vi "CalcTorqueFromJoint.vi"(8 "error in (no error)":errorcluster, 11 "CAlexData2 in":refnum<class "CAlex2_Data.lvclass">) -> (0 "error out":errorcluster, 1 "AverageTorque":T1, 2 "Torques":T2, 3 "CarexMData out":refnum<class "CAlex2_Data.lvclass">, 4 "Jacobian for Cables":dbl[][](array[numeric]))   [LabVIEW 2016, in "CAlex2_Data.lvclass"]
uses:
  CAlex2-Data/CAlex2_Data.lvclass
  C:/Users/Rand/Desktop/Bilateral-controller/CAlex2-controller/Sim&Process/DataProcess/ExpData/ExpData.lvclass
  <vilib>/Analysis/3filter.llb/Filter Passband Type.ctl
  CAlex2-Data/CAlex2_Data.lvclass/CAlex2_Data.ctl
  <vilib>/Analysis/baseanly.llb/A x Vector.vi
  Classes/CAlex2/CAlex2.lvclass
  C:/Users/Rand/Desktop/Bilateral-controller/CAlex2-controller/Classes/SerialChain/SerialChain.lvclass
  C:/Users/Rand/Desktop/Bilateral-controller/CAlex2-controller/Classes/SerialChain-Cable/SerialChain-Cable.lvclass
  Classes/SerialChain/SerialChain.lvclass
  Classes/SerialChain-Cable/SerialChain-Cable.lvclass
  <vilib>/Analysis/NI_AALBase.lvlib
  ExpData/ExpData.lvclass
  <vilib>/AuZn/auzn custom VIs/AuZnCustomVI.lvlib
panel:
  out "Numeric":i32
  out "PlannedTorque":dbl[][](array[numeric])
  out "ActualTorque":dbl[][](array[numeric])
  out "DesiredTorque":dbl[][](array[numeric])
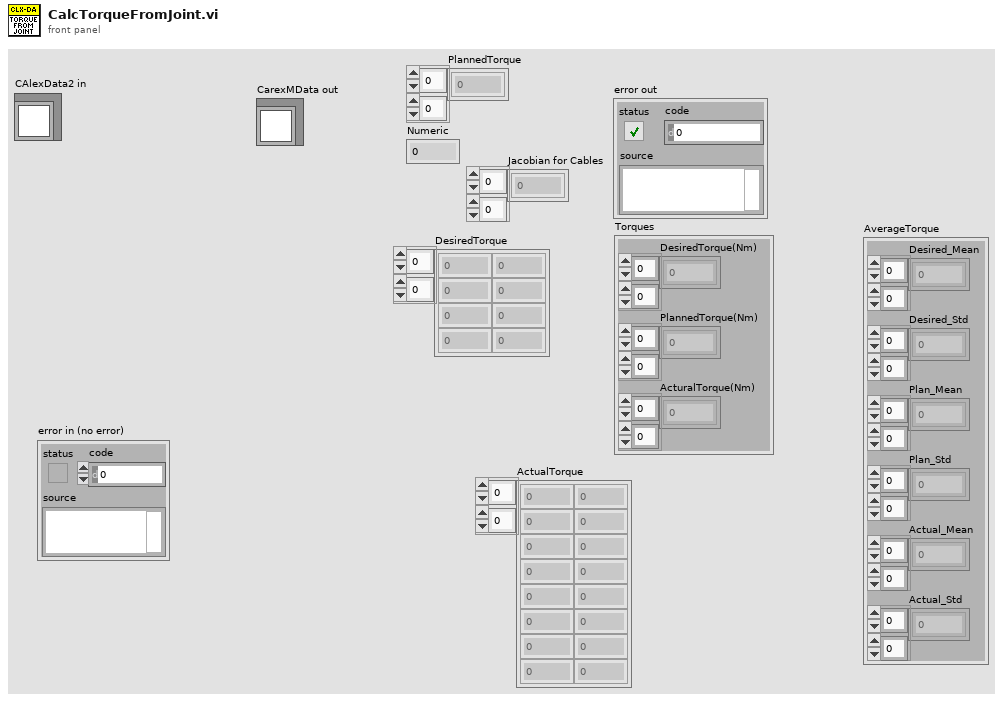
[diagram p1: front panel]
types:
  T1 = cluster{"Desired_Mean":dbl[][], "Desired_Std":dbl[][], "Plan_Mean":dbl[][], "Plan_Std":dbl[][], "Actual_Mean":dbl[][], "Actual_Std":dbl[][]}
  T2 = cluster{"DesiredTorque(Nm)":dbl[][], "PlannedTorque(Nm)":dbl[][], "ActuralTorque(Nm)":dbl[][]}
  T3 = typedef "NI_AALBase.lvlib/Filter Passband Type.ctl" = enum32{"Lowpass", "Highpass", "Bandpass", "Bandstop"}
  T4 = typedef "SerialChain.lvclass/PointOnBody.ctl" = cluster{"Coord4":dbl[], "ID":i32}
  T5 = typedef "NI_Matrix.lvlib/RealMatrix.ctl" = dbl[][]
  T6 = cluster{"Mean":dbl[][], "Std":dbl[][], "Mean":dbl[][], "Std":dbl[][], "Mean":dbl[][], "Std":dbl[][]}
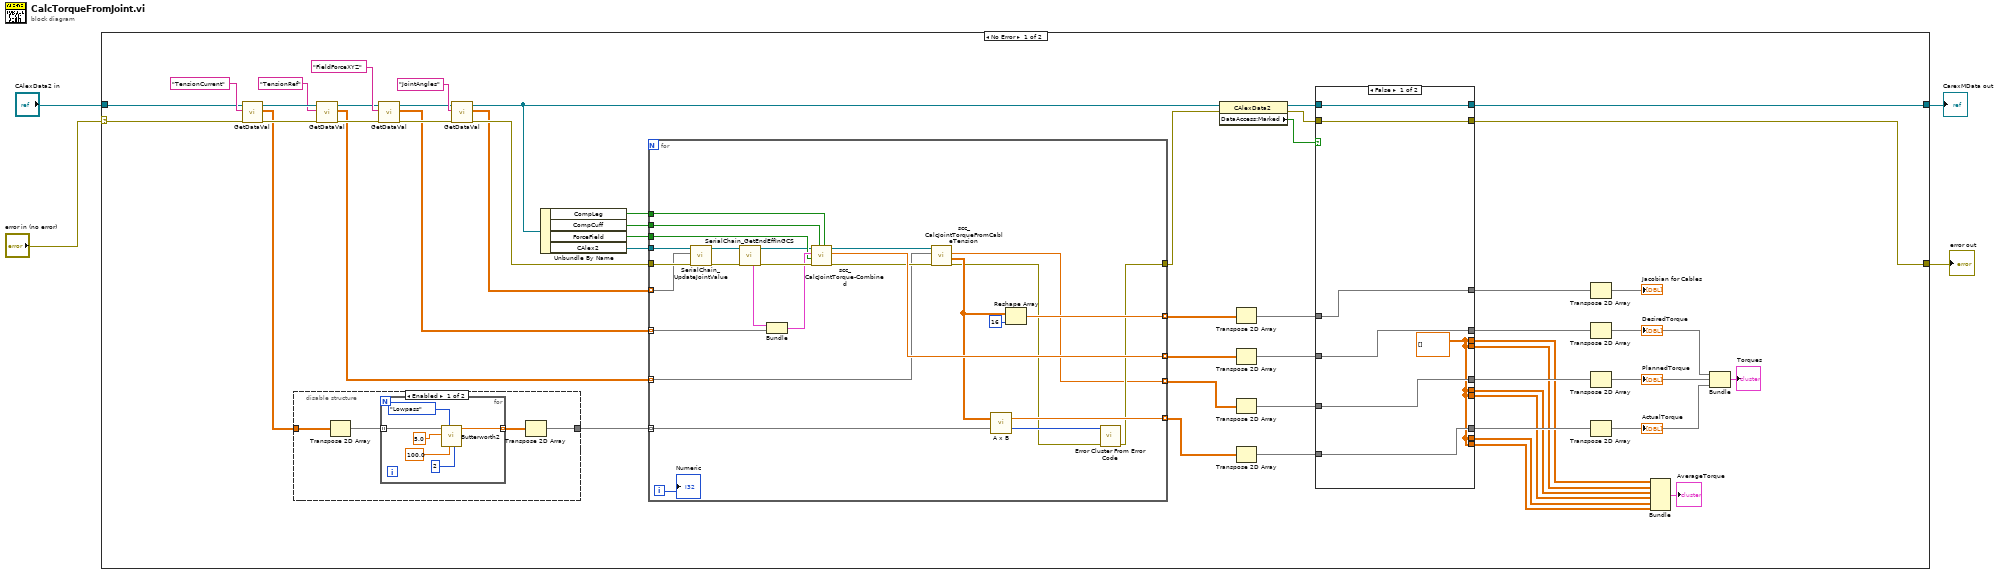
[diagram p0: block diagram]
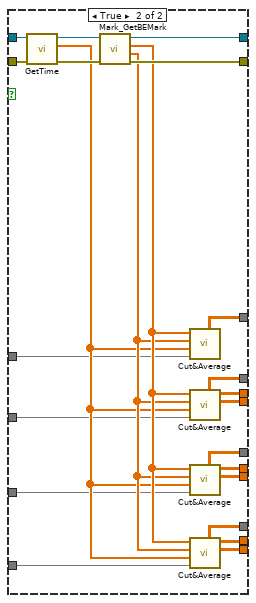
[diagram p2: hidden frame]
diagram:
  n1 = case shown="No Error" "error in (no error)" {
    selector: "error in (no error)" -> [w41 w126]
    tunnel: [w22 w126] -> w4
    tunnel: "CAlexData2 in" -> [w42 w127]
    tunnel: [w24 w127] -> w2
    frame No Error {
      n2 = call "GetDataVal.vi"("error in (no error)"=w41, "Name"="TensionCurrent", "ExpData in"=w42) -> ("error out"=w48:errorcluster, "Data"=w6:dbl[][], "ExpData out"=w50:refnum<class "CAlex2_Data.lvclass">)  [unwired: 5 in, 1 out]
      n3 = disable-structure shown="Enabled" {
        disable-tunnel: w6 -> [w90 w98]
        disable-tunnel: [w88 w98] -> w5
        frame Enabled {
          n4 = Transpose 2D Array(2D array=w90) -> (transposed array=w89:dbl[][])
          n5 = for {
            tunnel: w89 -> [w97] mode=indexing
            tunnel: [w96] -> w91 mode=indexing
            n6 = call <vilib>:"Butterworth2.vi"("order"=2, "sampling freq: fs"=100.0, "filter type"=Filter_Passband_Type."Lowpass", "low cutoff freq: fl"=5.0, "X"=w97) -> ("Filtered X"=w96:dbl[])  [unwired: 5 in, 1 out]
          }
          n7 = Transpose 2D Array(2D array=w91) -> (transposed array=w88:dbl[][])
        }
        frame Disabled {
        }
      }
      n8 = call "GetDataVal.vi"("error in (no error)"=w48, "Name"="TensionRef", "ExpData in"=w50) -> ("error out"=w47:errorcluster, "Data"=w37:dbl[][], "ExpData out"=w49:refnum<class "CAlex2_Data.lvclass">)  [unwired: 5 in, 1 out]
      n9 = call "GetDataVal.vi"("error in (no error)"=w47, "Name"="FieldForceXYZ", "ExpData in"=w49) -> ("error out"=w52:errorcluster, "Data"=w38:dbl[][], "ExpData out"=w53:refnum<class "CAlex2_Data.lvclass">)  [unwired: 5 in, 1 out]
      n10 = call "GetDataVal.vi"("error in (no error)"=w52, "Name"="JointAngles", "ExpData in"=w53) -> ("error out"=w40:errorcluster, "Data"=w39:dbl[][], "ExpData out"=w25:refnum<class "CAlex2_Data.lvclass">)  [unwired: 5 in, 1 out]
      n11 = Unbundle By Name(w25) -> ("CompLeg"=w44:bool, "CompCuff"=w45:bool, "ForceField"=w43:bool, "CAlex2"=w57:refnum<class "CAlex2.lvclass">)
      n12 = for {
        tunnel: w38 -> [w119] mode=indexing
        tunnel: [w118] -> w32 mode=indexing
        tunnel: [w117] -> w33 mode=indexing
        tunnel: w39 -> [w115] mode=indexing
        tunnel: w5 -> [w109] mode=indexing
        tunnel: [w114] -> w30 mode=indexing
        tunnel: [w108] -> w31 mode=indexing
        tunnel: w40 -> [w120]
        tunnel: [w112] -> w23
        tunnel: w57 -> [w99]
        tunnel: w37 -> [w105] mode=indexing
        tunnel: w45 -> [w104]
        tunnel: w44 -> [w103]
        tunnel: w43 -> [w102]
        i -> [w101]
        n13 = call "SerialChain_UpdateJointValue.vi"("error in (no error)"=w120, "JointAngle (rad | m)"=w115, "SerialChain in"=w99) -> ("error out"=w124:errorcluster, "SerialChain out"=w125:refnum<class "CAlex2.lvclass">)  [unwired: 7 in]
        n14 = call "SerialChain_GetEndEffInGCS.vi"("error in (no error)"=w124, "SerialChain in"=w125) -> ("error out"=w123:errorcluster, "SerialChain out"=w100:refnum<class "CAlex2.lvclass">, "EndEffPos"=w121:T4)  [unwired: 5 in, 2 out]
        n15 = Bundle("EndEffPos"=w121, "Data"=w119) -> (w122:cluster{"EndEffPos":T4, "Data":dbl[]})  [unwired: 1 in]
        n16 = call "scc_CalcJointTorque-Combined.vi"("BodyWtComp?(F)"=w103, "CuffWtComp?(T)"=w104, "error in (no error)"=w123, "ExternalForce(T)"=w102, "External Force (In GCS)"=w122, "SerialChain_Cable in"=w100) -> ("error out"=w110:errorcluster, "DesiredTorque(Nm)"=w118:dbl[], "SerialChain_Cable out"=w111:refnum<class "CAlex2.lvclass">)  [unwired: 3 in]
        n17 = call "scc_CalcJointTorqueFromCableTension.vi"("error in (no error)"=w110, "Cable Tensions"=w105, "SerialChain_Cable in"=w111) -> ("error out"=w106:errorcluster, "Jacobian for Cables"=w107:T5, "Joint Torque"=w108:dbl[])  [unwired: 5 in, 1 out]
        n18 = call-poly <vilib>:"A x B.vi"("Vector"=w109, "A"=w107) -> ("error"=w113:i32, "A x Vector"=w114:dbl[])
        n19 = Reshape Array(w107, 16 ("dimension size")) -> (w117:dbl[])
        n20 = call <vilib>:"Error Cluster From Error Code.vi"("error in (no error)"=w106, "error code (0)"=w113) -> ("error out"=w112:errorcluster)  [unwired: 7 in]
        "Numeric" <- w101
      }
      n21 = property class="CAlexData2"(reference=w25, error in=w23) -> (reference out=w36:refnum<class "CAlex2_Data.lvclass">, error out=w34:errorcluster, "DataAccess:Marked"=w35:bool)
      n22 = Transpose 2D Array(2D array=w33) -> (transposed array=w14:dbl[][])
      n23 = Transpose 2D Array(2D array=w32) -> (transposed array=w13:dbl[][])
      n24 = Transpose 2D Array(2D array=w31) -> (transposed array=w12:dbl[][])
      n25 = Transpose 2D Array(2D array=w30) -> (transposed array=w11:dbl[][])
      n26 = case shown="False" w35 {
        tunnel: w36 -> [w64 w85]
        tunnel: w34 -> [w63 w84]
        tunnel: [w63 w83] -> w22
        tunnel: [w64 w82] -> w24
        tunnel: [w59 w81] -> w26
        tunnel: [w60 w80] -> w27
        tunnel: [w61 w79] -> w28
        tunnel: [w62 w78] -> w29
        tunnel: w14 -> [w62 w74]
        tunnel: w13 -> [w61 w73]
        tunnel: w12 -> [w60 w72]
        tunnel: w11 -> [w59 w71]
        tunnel: [w58 w70] -> w21
        tunnel: [w58 w69] -> w20
        tunnel: [w58 w68] -> w19
        tunnel: [w58 w67] -> w18
        tunnel: [w58 w66] -> w17
        tunnel: [w58 w65] -> w16
        frame False {
          w58 = dbl[][] [] ("Mean")
        }
        frame True {
          n27 = call "GetTime.vi"("error in (no error)"=w84, "ExpData in"=w85) -> ("error out"=w87:errorcluster, "Time"=w75:dbl[], "ExpData out"=w86:refnum<class "CAlex2_Data.lvclass">)  [unwired: 7 in]
          n28 = call "Mark_GetBEMark.vi"("error in (no error)"=w87, "ExpData In"=w86) -> ("error out"=w83:errorcluster, "End"=w76:dbl[], "Begin"=w77:dbl[], "ExpData Out"=w82:refnum<class "CAlex2_Data.lvclass">)  [unwired: 5 in, 1 out]
          n29 = call <vilib>:"Cut&Average.vi"("Data"=w74, "Time"=w75, "End"=w76, "Begin"=w77) -> ("CuttedData-Concatenated"=w78:dbl[][])  [unwired: 2 in, 5 out]
          n30 = call <vilib>:"Cut&Average.vi"("Data"=w73, "Time"=w75, "End"=w76, "Begin"=w77) -> ("Std"=w69:dbl[][], "Mean"=w70:dbl[][], "CuttedData-Concatenated"=w79:dbl[][])  [unwired: 2 in, 3 out]
          n31 = call <vilib>:"Cut&Average.vi"("Data"=w72, "Time"=w75, "End"=w76, "Begin"=w77) -> ("Std"=w67:dbl[][], "Mean"=w68:dbl[][], "CuttedData-Concatenated"=w80:dbl[][])  [unwired: 2 in, 3 out]
          n32 = call <vilib>:"Cut&Average.vi"("Data"=w71, "Time"=w75, "End"=w76, "Begin"=w77) -> ("Std"=w65:dbl[][], "Mean"=w66:dbl[][], "CuttedData-Concatenated"=w81:dbl[][])  [unwired: 2 in, 3 out]
        }
      }
      n33 = Transpose 2D Array(2D array=w29) -> (transposed array=→"Jacobian for Cables":dbl[][])
      n34 = Transpose 2D Array(2D array=w28) -> (transposed array=w9:dbl[][])
      "DesiredTorque" <- w9
      n35 = Transpose 2D Array(2D array=w27) -> (transposed array=w8:dbl[][])
      "PlannedTorque" <- w8
      n36 = Transpose 2D Array(2D array=w26) -> (transposed array=w7:dbl[][])
      "ActualTorque" <- w7
      n37 = Bundle("Mean"=w21, "Std"=w20, "Mean"=w19, "Std"=w18, "Mean"=w17, "Std"=w16) -> (→"AverageTorque":T6)  [unwired: 1 in]
      n38 = Bundle(w9, w8, w7) -> (→"Torques":cluster{dbl[][], dbl[][], dbl[][]})  [unwired: 1 in]
    }
    frame Error {
    }
  }
  "error out" <- w4
  "CarexMData out" <- w2
